vi "Get 3D Live Position Offset.vi"(3 "Mode":T5, 5 "Traverse line In":T2 {"Carrier_2 Q (l/min)" format="%#.2f"; "Row Duration (mins)" format="%#.1f"; "Row No" min=0; "Trace Gas Concentration (%)" min=0.0 format="%#_4f"; "Carrier_1 Q (l/min)" format="%#.4f"; "Tunnel Speed" format="%#.2f"; "Start X" format="%#.2f"; "Start Y" format="%#.2f"; "Start Z" format="%#.2f"; "End X" format="%#.2f"; "End Y" format="%#.2f"; "End Z" format="%#.2f"; "Averaging time (min)" min=0.0 format="%#.2f"}) -> (0 "Error Message":string, 1 "Status":T1, 2 "Traverse line Out":T2 {"Carrier_2 Q (l/min)" format="%#.2f"; "Row Duration (mins)" format="%#.1f"; "Row No" min=0; "Trace Gas Concentration (%)" min=0.0 format="%#_4f"; "Carrier_1 Q (l/min)" format="%#.4f"; "Tunnel Speed" format="%#.2f"; "Start X" format="%#.2f"; "Start Y" format="%#.2f"; "Start Z" format="%#.2f"; "End X" format="%#.2f"; "End Y" format="%#.2f"; "End Z" format="%#.2f"; "Averaging time (min)" min=0.0 format="%#.2f"})   [LabVIEW 2020]
uses:
  Controls/Setup.ctl
  Controls/Save_Data.ctl
  Globals/Meas_global.vi
  Globals/Trav_pos_global.vi
  Gen Trav/Multi_Run_Status.ctl
  Controls/User_Specific_mode.ctl
  Globals/Extra_Commands_Global.vi
  Globals/Dynamic_call_global.ph.vi
  Globals/Preference_global.vi
  Gen Trav/Spacing.ctl
  Gen Trav/Traverse_cluster.ctl
  Controls/Multi_run_mode.ctl
panel:
  out "Offsets":sgl[](array[numeric])
  # "X            Y              Z"
  # "X           Y            Z"
  # "Start"
  # "End"
  # "X           Y            Z"
  # "Start"
  # "End"
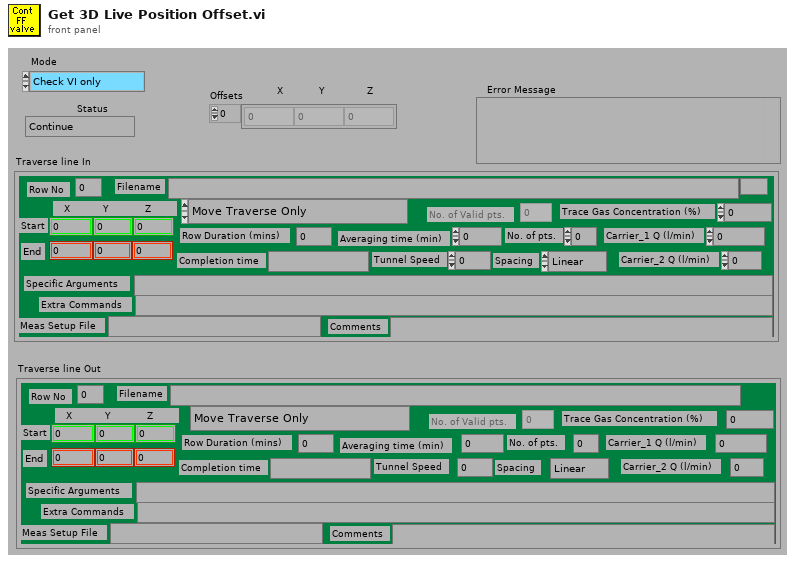
[diagram p1: front panel]
types:
  T1 = typedef "Multi_Run_Status.ctl" = enum16{"Continue", "Continue with Error", "Jump to Next Point", "Jump to Next Row", "Jump To Fall Back", "Terminate Run"}
  T2 = typedef "Traverse_cluster.ctl" = cluster{"Start X":sgl, "Start Y":sgl, "Start Z":sgl, "End X":sgl, "End Y":sgl, "End Z":sgl, "No. of pts.":i32, "Spacing":T3, "Filename":path, "Tunnel Speed":dbl, "Averaging time (min)":dbl, "Extra Commands":string, "Carrier_1 Q (l/min)":dbl, "Carrier_2 Q (l/min)":dbl, "Trace Gas Concentration (%)":dbl, "Specific Arguments":string, "Comments":string, "Row No":i32, "Row Type Selector":T4, "Completion time":string, "Row Duration (mins)":dbl, "No. of Valid pts.":i32, "Meas Setup File":string}
  T3 = typedef "Spacing.ctl" = enum16{"Linear", "Log", "Gauss", "Specified", "N/A"}
  T4 = typedef "Multi_run_mode.ctl" = enum16{"Move Traverse Only", "Set Tunnel Speed Only", "Set Source Only", "Set Measurement Conditions", "Single Measurement", "Vertical Profile", "Lateral Profile", "Longitudinal Profile", "Multi-Axis Profile", "Explore Volume", "Auto Calibrate", "Meas Fast FID Bkgnd", "Check Beam Power", "Scanning Valve Measurement", "Run VI Named:", "Set ADAM Ch", "Wait (minutes)", "Send Message", "Synchronize With:", "Fall Back to this Row", "Turn Off Row Repeating", "Traverse 3D Volume", "Blank Row", "Jump to Fall Back Row"}
  T5 = typedef "User_Specific_mode.ctl" = enum16{"Check VI only", "Run VI"}
  T6 = typedef "Save_Data.ctl" = enum16{"Save No Data", "Save Data"}
  T7 = typedef "Setup.ctl" = enum16{"Run Program", "Show Setup", "Save Current Setup", "Setup Front Panel"}
  T8 = typedef "Status_Cluster.ctl" = cluster{"Status":T1, "Error Type":string, "Error Description":string}
  T9 = typedef "Analysis_info_cluster.ctl" = cluster{"Colour":u32, "Inst type":T10, "Inst name":string, "Symbol":string, "Code name":string, "Extra Info":string, "Inst Array":T11, "Extra Titles":string[], "Extra Values":string[], "U":dbl, "u^2":dbl, "u^3":dbl, "u^4":dbl, "Skew_u":dbl, "Kurt_u":dbl, "Sd Error in Mean":dbl, "% u'/U":dbl, "X":dbl, "Y":dbl, "Z":dbl, "Timescale integral Estimate":dbl, "Sd Error in Variance":dbl, "Calib File":path, "Calib Constants":dbl[], "Output Position":bool, "Stats":enum16{"None", "Basic", "Full"}, "Av Sampling Rate":dbl, "Av No of Samples":dbl, "Total Meas Time (s)":dbl, "ADAM Ch Name":string, "Max value":dbl, "Min value":dbl, "Req Sample Rate Hz":dbl, "Sync Delay Time (s)":dbl, "Ch No":i16, "Device":string, "Use Latest Calib":bool, "Port":string, "Metadata Ch Names":string[], "Metadata Ch Values":string[], "Label":string}
  T10 = typedef "Inst_type.ctl" = enum16{"Propeller anemometer", "Raw voltage", "Pressure Transducer", "Pitot-static tube", "Hot wire", "Cross wire 1", "Cross wire 2", "Generic Linear", "Generic Polynomial", "Generic BackPoly", "Fast FID", "Thermocouple", "Cold wire", "Pulsed Wire", "LDA Vel", "LDA Tran time", "LDA Arr time", "Microphone"}
  T11 = typedef "Instrument_Array.ctl" = enum16{"PWA", "LDA", "Analogue"}
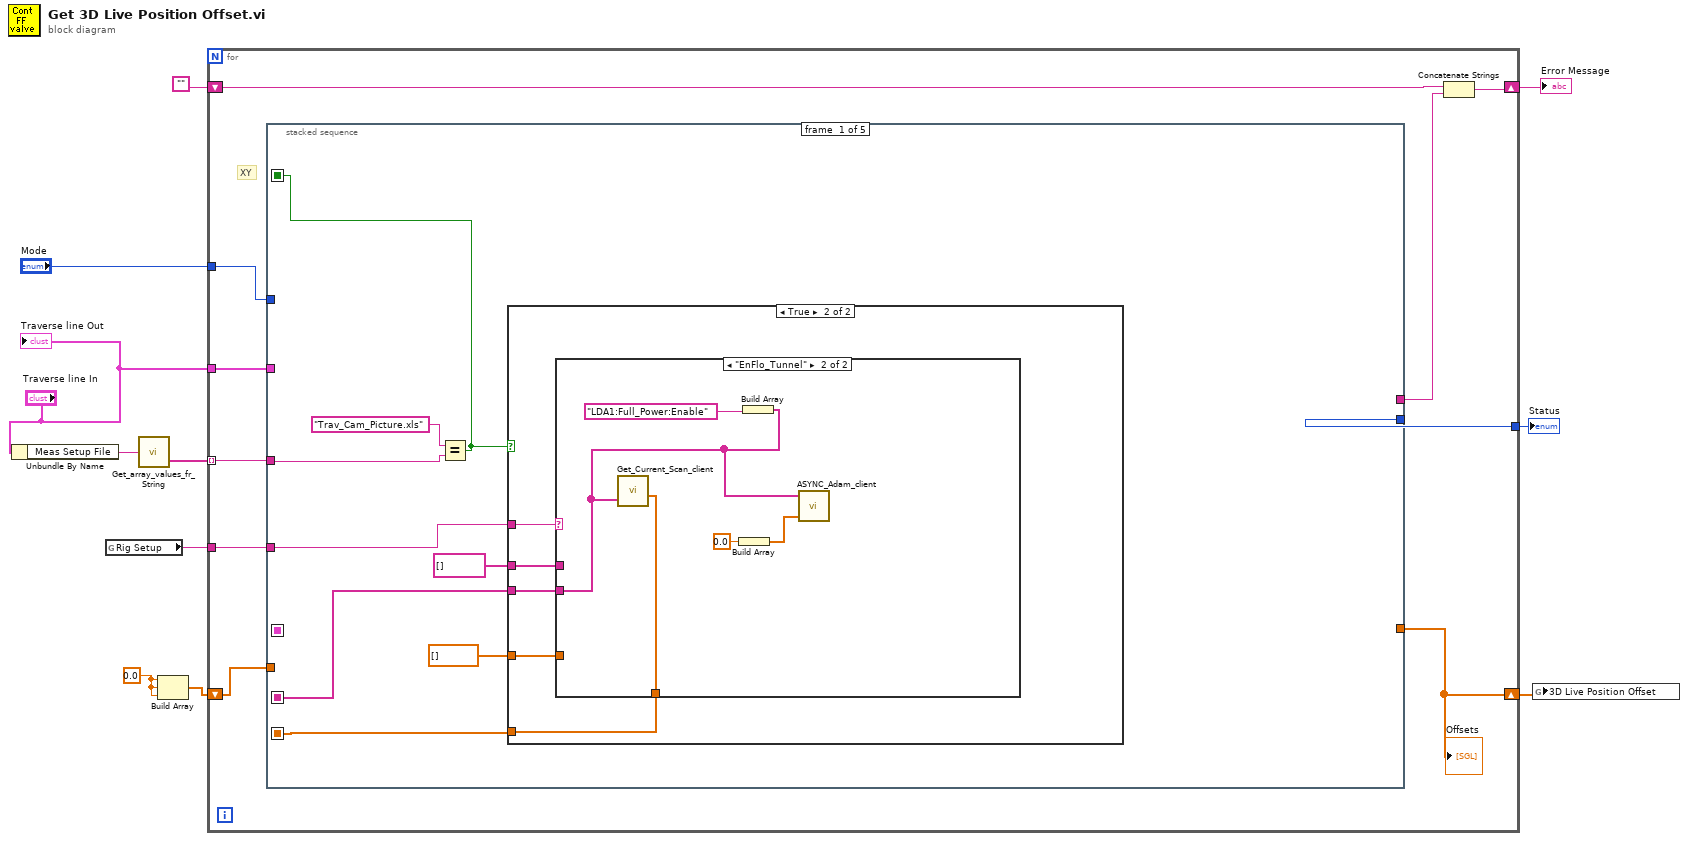
[diagram p0: block diagram]
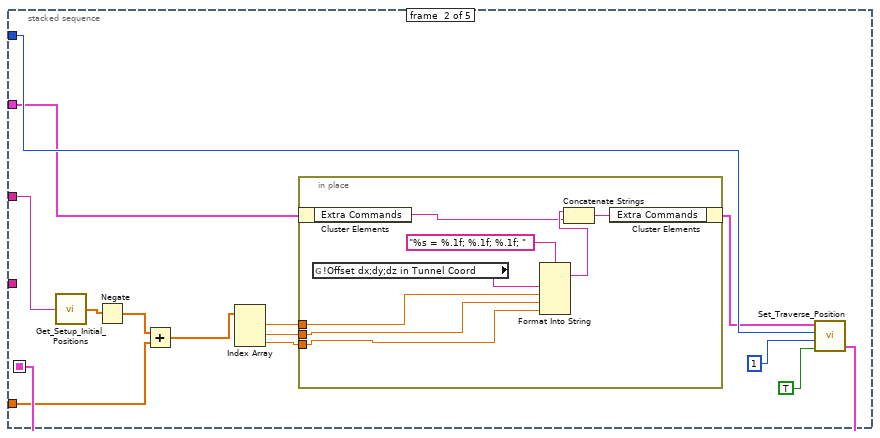
[diagram p4: hidden frame]
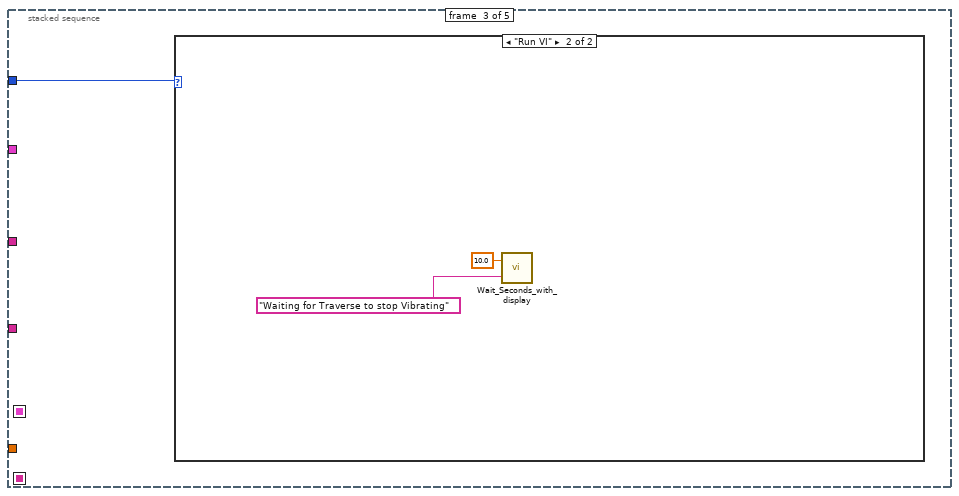
[diagram p5: hidden frame]
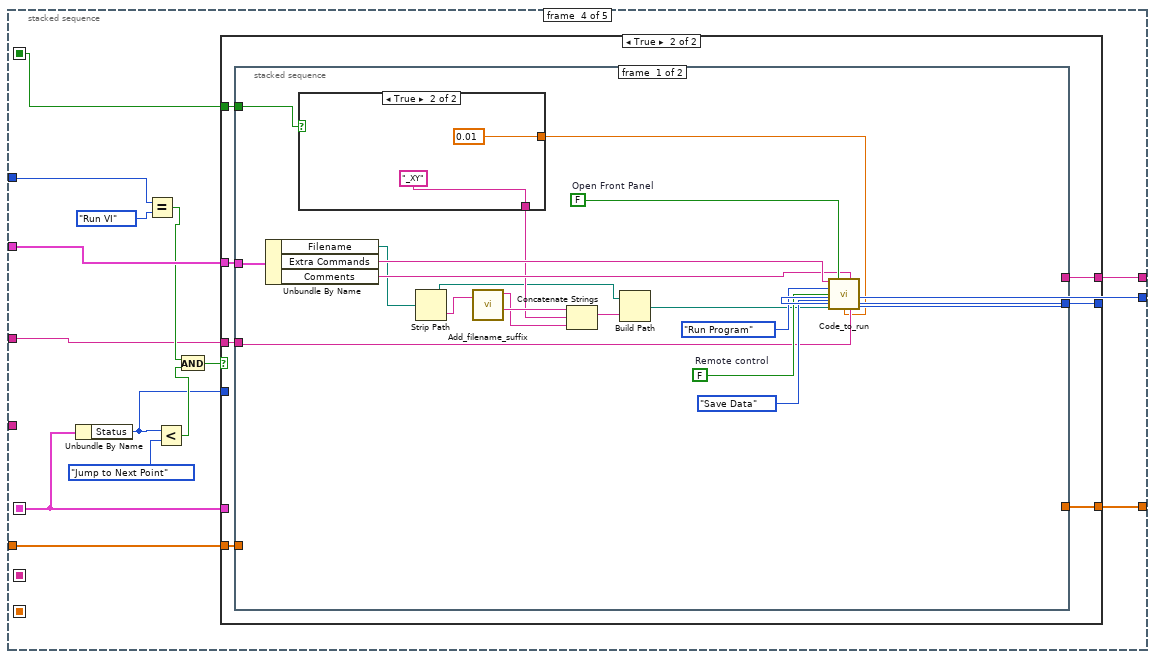
[diagram p7: hidden frame]
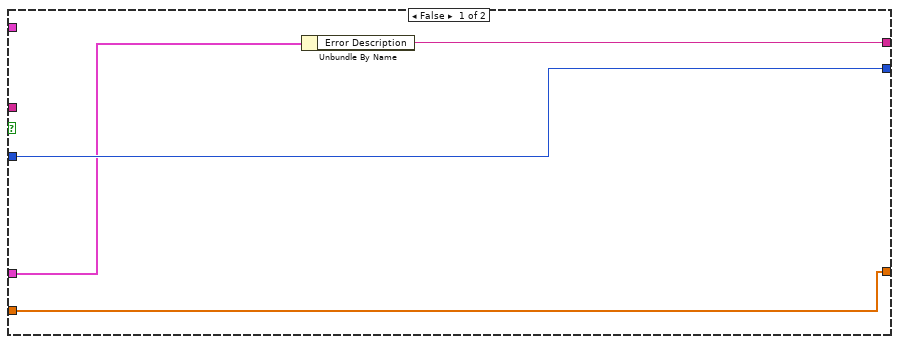
[diagram p8: hidden frame]
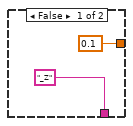
[diagram p9: hidden frame]
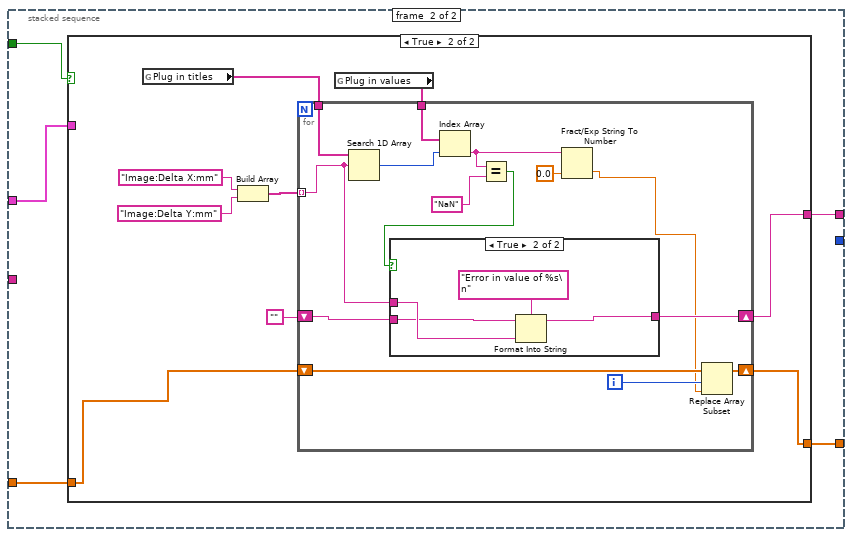
[diagram p10: hidden frame]
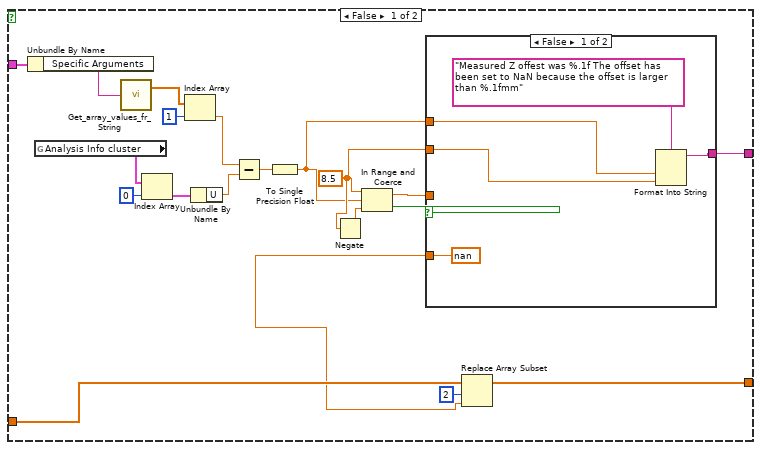
[diagram p11: hidden frame]
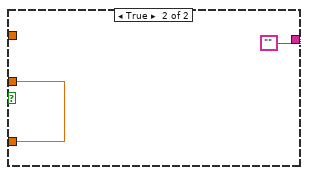
[diagram p12: hidden frame]
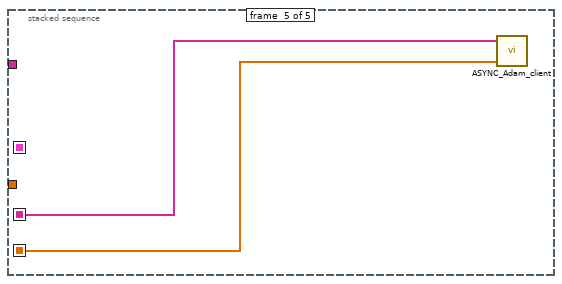
[diagram p14: hidden frame]
diagram:
  w4 = sgl 0.0
  n1 = Unbundle By Name("Traverse line In") -> ("Meas Setup File"=w9:string)
  n2 = global read "Preference_global.vi" "Rig Setup"() -> (w1:string)
  n3 = call "Get_array_values_fr_String.vi"("String Value"=w9) -> ("String array"=w8:string[])  [unwired: 1 out]
  n4 = Build Array(w4, w4, w4) -> (w3:sgl[])
  n5 = for {
    tunnel: "Mode" -> [w21]
    tunnel: "Traverse line In" -> [w19]
    tunnel: w8 -> [w18] mode=indexing
    tunnel: [w17] -> w7
    shift-right: [w15] -> w5
    shift-left: "" -> [w16]
    shift-right: [w13] -> w2
    shift-left: w3 -> [w14]
    tunnel: w1 -> [w12]
    # "XY"
    n6 = stacked-sequence {
      seq-local: [_ w54 _ _ _] -> [_ _ _ w73 _]
      seq-local: [w26 _ _ _ _] -> [_ _ _ w69 _]
      seq-local: [w25 _ _ _ _] -> [_ _ _ _ w179]
      seq-local: [w22 _ _ _ _] -> [_ _ _ _ w178]
      tunnel: [_ _ _ w74 _] -> w20
      tunnel: w19 -> [_ w53 _ w83 _]
      tunnel: w21 -> [_ w55 w66 w80 _]
      tunnel: [_ _ _ w76 _] -> w17
      tunnel: w18 -> [w28 w48 _ w72 _]
      tunnel: w14 -> [_ w46 _ w71 _]
      tunnel: [_ _ _ w70 _] -> w13
      tunnel: w12 -> [w27 _ _ _ _]
      frame #0 {
        n7 = Equal?(x="Trav_Cam_Picture.xls", y=w28) -> (x = y?=w26:bool)
        n8 = case shown="True" w26 {
          tunnel: w27 -> [_ w36]
          tunnel: [w31 w34] -> w22
          tunnel: [w30 w32] -> w25
          tunnel: dbl[] [] ("Numerical Values") -> [w30 w33]
          tunnel: string[] [] -> [w31 w35]
          frame False {
          }
          frame True {
            n9 = case shown="\"EnFlo_Tunnel\"" w36 {
              tunnel: [w38 w39] -> w34
              tunnel: [w37 w41] -> w32
              tunnel: w35 -> [w38 _]
              tunnel: w33 -> [w37 _]
              frame Default {
              }
              frame "EnFlo_Tunnel" {
                n10 = Build Array(0.0 ("element")) -> (w42:dbl[])
                n11 = Build Array("LDA1:Full_Power:Enable") -> (w39:string[])
                n12 = call "Get_Current_Scan_client.vi"("multipleChannels"=w39) -> ("Numerical Values"=w41:dbl[])  [unwired: 2 in, 2 out]
                n13 = call "ASYNC_Adam_client.vi"("Values"=w42, "Channel Names"=w39) -> ()  [unwired: 1 in, 2 out]
              }
            }
          }
        }
      }
      frame #1 {
        n14 = call "Get_Setup_Initial_Positions.vi"("Setup Filename"=w48) -> ("Initial Offsets"=w47:sgl[])
        n15 = Negate(x=w47) -> (-x=w45:sgl[])
        n16 = Add(x=w45, y=w46) -> (x+y=w44:sgl[])
        n17 = Index Array(array=w44) -> (element #1=w51:sgl, element #2=w50:sgl, element #3=w49:sgl)  [unwired: 3 in]
        n18 = in-place {
          in-place-border: w51 -> [w60]
          in-place-border: w50 -> [w59]
          in-place-border: w49 -> [w58]
          n19 = in-place-cluster #1(w53) -> ("Extra Commands"=w62:string)
          n20 = global read "Extra_Commands_Global.vi" "!Offset dx;dy;dz in Tunnel Coord"() -> (w64:string)
          n21 = Format Into String(format string="%s = %.1f; %.1f; %.1f; ", w64, w60, w59, w58) -> (resulting string=w63:string)  [unwired: 2 in, 1 out]
          n22 = Concatenate Strings(w63, w62) -> (w61:string)
          n23 = in-place-cluster #1("Extra Commands"=w61) -> (w52:T2)
        }
        n24 = call "Set_Traverse_Position.vi"("Last Part of Move?"=TRUE, "Currently on Point"=1, "Simulate/Run"=w55, "Traverse line"=w52) -> ("Status Cluster"=w54:T8)  [unwired: 2 in]
      }
      frame #2 {
        n25 = case shown="\"Run VI\"" w66 {
          frame "Check VI only", Default {
          }
          frame "Run VI" {
            n26 = call "Wait_Seconds_with_display.vi"("Message"="Waiting for Traverse to stop Vibrating", "Seconds to wait"=10.0) -> ()  [unwired: 1 in, 1 out]
          }
        }
      }
      frame #3 {
        n27 = Unbundle By Name(w73) -> ("Status"=w75:T1)
        n28 = Equal?(x=w80, y=User_Specific_mode."Run VI" ("Mode")) -> (x = y?=w78:bool)
        n29 = Less?(x=w75, y=Multi_Run_Status."Jump to Next Point") -> (x < y?=w79:bool)
        n30 = And(x=w78, y=w79) -> (x .and. y?=w77:bool)
        n31 = case shown="True" w77 {
          tunnel: [w87 w94] -> w76
          tunnel: w83 -> [_ w93]
          tunnel: w75 -> [w87 _]
          tunnel: [w85 w92] -> w74
          tunnel: w73 -> [w86 _]
          tunnel: w72 -> [_ w91]
          tunnel: w71 -> [w84 w90]
          tunnel: [w84 w89] -> w70
          tunnel: w69 -> [_ w88]
          frame False {
            n32 = Unbundle By Name(w86) -> ("Error Description"=w85:string)
          }
          frame True {
            n33 = stacked-sequence {
              tunnel: [w113 _] -> w94
              tunnel: w93 -> [w106 w122]
              tunnel: [_ w121] -> w92
              tunnel: w91 -> [w105 _]
              tunnel: w90 -> [_ w120]
              tunnel: [_ w119] -> w89
              tunnel: w88 -> [w95 w118]
              frame #0 {
                w111 = FALSE  # Open Front Panel
                w112 = FALSE  # Remote control
                n34 = Unbundle By Name(w106) -> ("Filename"=w103:path, "Extra Commands"=w108:string, "Comments"=w107:string)
                n35 = case shown="True" w95 {
                  tunnel: [0.1 ("Averaging time (min)") 0.01 ("Averaging time (min)")] -> w104
                  tunnel: ["_Z" "_XY"] -> w100
                  frame False {
                  }
                  frame True {
                  }
                }
                n36 = Strip Path(path=w103) -> (stripped path=w97:path, name=w102:string)
                n37 = call "Add_filename_suffix.vi"("Filename"=w102) -> ("Original Suffix"=w99:string, "Base name"=w101:string)  [unwired: 1 in, 2 out]
                n38 = Concatenate Strings(w101, w100, w99) -> (w98:string)
                n39 = Build Path(base path=w97, name or relative path=w98) -> (appended path=w96:path)
                n40 = call "Code_to_run.vi"("Extra command String"=w108, "Open Front Panel"=w111, "Current Row Comments"=w107, "setup"=Setup."Run Program", "Remote control"=w112, "File"=Save_Data."Save Data", "Results Filename"=w96, "Averaging time (min)"=w104, "Setup filename"=w105) -> ("Status"=w113:T1)  [unwired: 3 in, 3 out]
              }
              frame #1 {
                n41 = case shown="True" w118 {
                  tunnel: w122 -> [w129 _]
                  tunnel: [w128 w152] -> w121
                  tunnel: w120 -> [w126 w151]
                  tunnel: [w123 w150] -> w119
                  frame False {
                    w130 = sgl 8.5 ("upper limit")
                    n42 = Unbundle By Name(w129) -> ("Specific Arguments"=w139:string)
                    n43 = global read "Meas_global.vi" "Analysis Info cluster"() -> (w142:T9[])
                    n44 = call "Get_array_values_fr_String.vi"("String Value"=w139) -> ("Numeric Array"=w137:dbl[])  [unwired: 1 out]
                    n45 = Index Array(array=w142, index=0) -> (element=w140:T9)
                    n46 = Index Array(array=w137, index=1) -> (element=w136:dbl)
                    n47 = Unbundle By Name(w140) -> ("U"=w135:dbl)
                    n48 = Subtract(x=w136, y=w135) -> (x-y=w134:dbl)
                    n49 = To Single Precision Float(number=w134) -> (single precision float=w127:sgl)
                    n50 = Negate(x=w130) -> (-x=w133:sgl)
                    n51 = In Range and Coerce(upper limit=w130, x=w127, lower limit=w133) -> (coerced(x)=w131:sgl, In Range?=w132:bool)
                    n52 = case shown="False" w132 {
                      tunnel: w127 -> [w147 _]
                      tunnel: w131 -> [_ w148]
                      tunnel: [w145 ""] -> w128
                      tunnel: [sgl nan ("upper limit") w148] -> w124
                      tunnel: w130 -> [w143 _]
                      frame False {
                        n53 = Format Into String(format string="Measured Z offest was %.1f The offset has  been set to NaN because the offset is larger than %.1fmm", w147, w143) -> (resulting string=w145:string)  [unwired: 2 in, 1 out]
                      }
                      frame True {
                      }
                    }
                    n54 = Replace Array Subset(array=w126, new element=w124, index=2) -> (w123:sgl[])
                  }
                  frame True {
                    n55 = global read "Dynamic_call_global.ph.vi" "Plug in titles"() -> (w157:string[])
                    n56 = Build Array("Image:Delta X:mm", "Image:Delta Y:mm") -> (w154:string[])
                    n57 = global read "Dynamic_call_global.ph.vi" "Plug in values"() -> (w158:string[])
                    n58 = for {
                      tunnel: w158 -> [w168]
                      tunnel: w157 -> [w167]
                      tunnel: w154 -> [w165] mode=indexing
                      shift-right: [w163] -> w152
                      shift-left: "" -> [w164]
                      shift-right: [w162] -> w150
                      shift-left: w151 -> [w161]
                      i -> [w160]
                      n59 = Search 1D Array(1D array=w167, element=w165) -> (index of element=w171:i32)  [unwired: 1 in]
                      n60 = Index Array(array=w168, index=w171) -> (element=w169:string)
                      n61 = Equal?(x=w169, y="NaN") -> (x = y?=w166:bool)
                      n62 = case shown="True" w166 {
                        tunnel: w165 -> [_ w176]
                        tunnel: w164 -> [w173 w175]
                        tunnel: [w173 w174] -> w163
                        frame False {
                        }
                        frame True {
                          n63 = Format Into String(format string="Error in value of %s\n", initial string=w175, w176) -> (resulting string=w174:string)  [unwired: 1 in, 1 out]
                        }
                      }
                      n64 = Fract/Exp String To Number(string=w169, default (0 dbl)=sgl 0.0 ("default (0 DBL)")) -> (number=w159:sgl)  [unwired: 2 in, 1 out]
                      n65 = Replace Array Subset(array=w161, new element=w159, index=w160) -> (w162:sgl[])
                    }
                  }
                }
              }
            }
          }
        }
      }
      frame #4 {
        n66 = call "ASYNC_Adam_client.vi"("Values"=w179, "Channel Names"=w178) -> ()  [unwired: 1 in, 2 out]
      }
    }
    "Offsets" <- w13
    n67 = Concatenate Strings(w16, w20) -> (w15:string)
  }
  "Status" <- w7
  "Error Message" <- w5
  n68 = global write "Trav_pos_global.vi" "3D Live Position Offset"(w2) -> ()
  "Traverse line Out" <- "Traverse line In"
